vi "StartTask.vi"(8 "error in (no error)":errorcluster, 10 "Task":string, 11 "DAQ_Module in":refnum<class "DAQ_Module.lvclass">) -> (0 "error out":errorcluster, 2 "daq error":errorcluster, 3 "DAQ_Module out":refnum<class "DAQ_Module.lvclass">)   [LabVIEW 2025, in "DAQ_Module.lvlib" / "DAQ_Module.lvclass"]
uses:
  DAQ_Module.lvclass
  DAQ_Module.lvclass/DAQ_Module.ctl
  <vilib>/ActorFramework/Message Enqueuer/Message Enqueuer.lvclass/Message Enqueuer.ctl
  <vilib>/ActorFramework/Message Enqueuer/Enqueue.vi
  DAQ_Abstr/Task_Abstr/Task_Abstr Messages/StartTask Msg/StartTask Msg.lvclass
  <vilib>/ActorFramework/Message Priority Queue/Priority Enqueue.vi
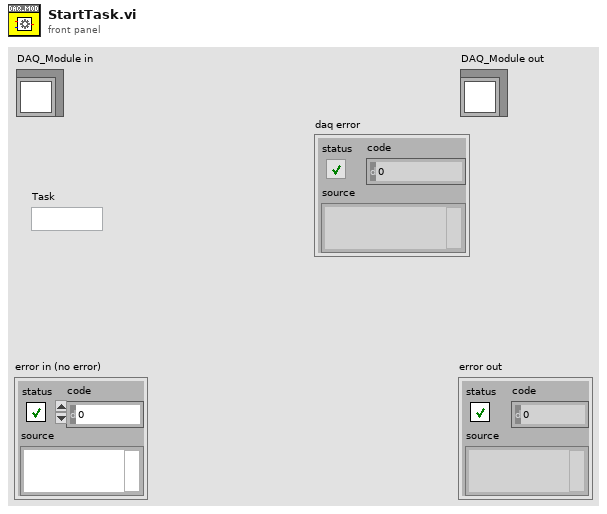
[diagram p1: front panel]
types:
  T1 = map{string, refnum<class "Message Enqueuer.lvclass">}
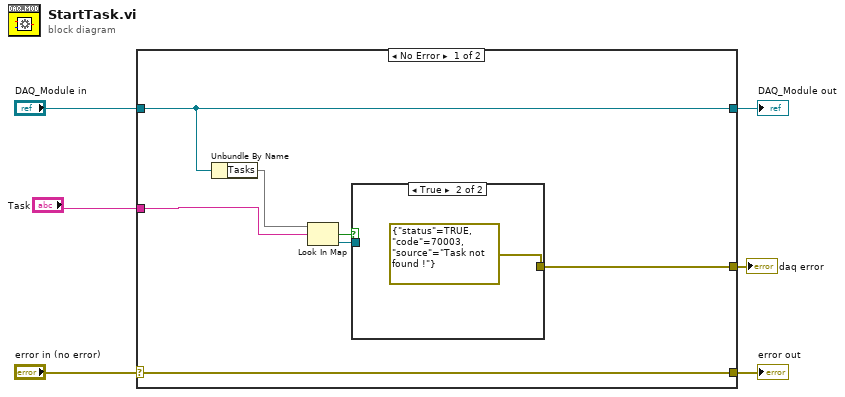
[diagram p0: block diagram]
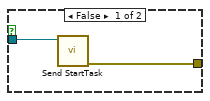
[diagram p2: hidden frame]
diagram:
  n1 = case shown="No Error" "error in (no error)" {
    selector: "error in (no error)" -> [w13 w18]
    tunnel: [w13 w18] -> w5
    tunnel: [w9 w17] -> w3
    tunnel: "DAQ_Module in" -> [w9 w17]
    tunnel: "Task" -> [w8 _]
    tunnel: [w7 _] -> w1
    frame No Error {
      n2 = Unbundle By Name(w9) -> ("Tasks"=w12:T1)
      n3 = Look In Map(map=w12, key=w8) -> (key not found?=w10:bool, value=w11:refnum<class "Message Enqueuer.lvclass">)  [unwired: 1 in]
      n4 = case shown="True" w10 {
        tunnel: w11 -> [w15 _]
        tunnel: [w14 errorcluster {"status"=TRUE, "code"=70003, "source"="Task not found !"} ("error out")] -> w7
        frame False {
          n5 = call "Send StartTask.vi"("Message Enqueuer"=w15) -> ("error out"=w14:errorcluster)  [unwired: 9 in, 1 out]
        }
        frame True {
        }
      }
    }
    frame Error {
    }
  }
  "error out" <- w5
  "DAQ_Module out" <- w3
  "daq error" <- w1
